vi "Set Actor Monitor.vi"(8 "error in (no error)":errorcluster, 10 "Actor Monitor":refnum<class "Actor Monitor.lvclass"> caption="Actor Monitor (Unwired = No Monitor)") -> (0 "error out":errorcluster)   [LabVIEW 2017, in "MGI-Monitored Actor Core.lvlib"]
doc: "Sets the type of actor monitor to use.\n----\nCopyright: MGI 2018\nAuthor: Derek Trepanier"
uses:
  MGI-Monitored Actor Core.lvlib
  Actor Monitor/Actor Monitor/Actor Monitor.lvclass
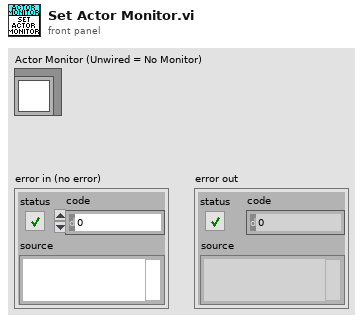
[diagram p1: front panel]
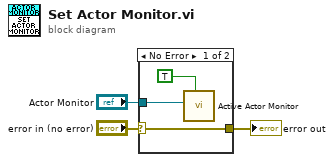
[diagram p0: block diagram]
diagram:
  n1 = case shown="No Error" "error in (no error)" {
    selector: "error in (no error)" -> [w4 w7]
    tunnel: "Actor Monitor" -> [w6 _]
    tunnel: [w4 w7] -> w1
    frame No Error {
      n2 = call "Active Actor Monitor.vi"("Write? (f)"=TRUE, "Monitor Type in"=w6) -> ()  [unwired: 9 in, 1 out]
    }
    frame Error {
    }
  }
  "error out" <- w1
